vi "Tx Message to Map Value.vi"(7 "parameter index":i32, 8 "error in":errorcluster, 9 "message":T2={"name"="", "message type"="BC to RT", "endpoint Tx"={"terminal address"=0, "subaddress"=0}, "endpoint Rx"={"terminal address"=0, "subaddress"=0}, "create timestamp channel"=FALSE, "mode code"=0, "number of words"=0, "parameters"=[]}, 10 "remote terminal handles":u64[](array[numeric]), 11 "bus controller handle":u64) -> (0 "error out":errorcluster, 3 "Tx write info":T1, 5 "next parameter index":i32)   [LabVIEW 2020, in "Ballard MIL-STD-1553 Engine.lvlib" / "Custom Device.lvlib"]
uses:
  Custom Device.lvlib
  Shared/Message Definition.ctl
  Shared/Message Type.ctl
  Shared/Terminal Endpoint.ctl
  Shared/Address.ctl
  Shared/Parameter Definition.ctl
  Shared/Tx Write Info.ctl
  <instrlib>/BTI1553Lib/Public/Controls/1553 RT Transfer Type.ctl
  <instrlib>/BTI1553Lib/Public/Controls/1553 Transfer Direction.ctl
  <instrlib>/BTI1553Lib/Private/RT/Configure/Get RT Xfer Handle.vi
  <instrlib>/BTI1553Lib/BTI1553LV.lvlib
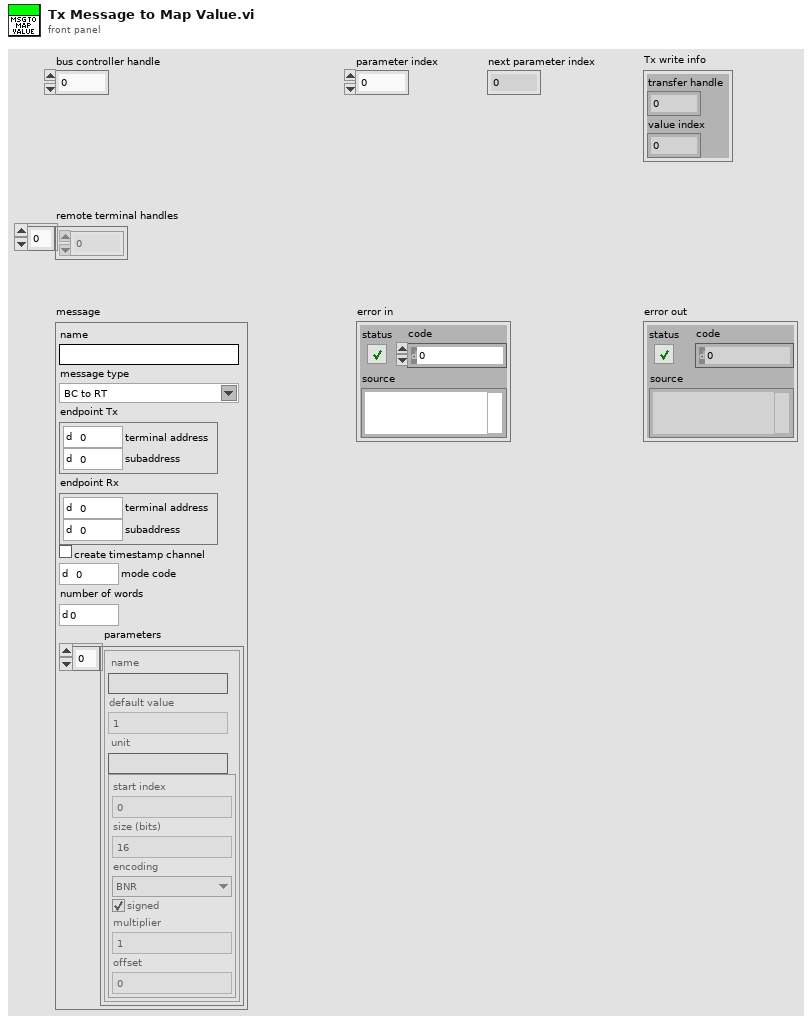
[diagram p1: front panel]
types:
  T1 = typedef "Tx Write Info.ctl" = cluster{"transfer handle":u64, "value index":i32}
  T2 = typedef "Message Definition.ctl" = cluster{"name":string, "message type":T3, "endpoint Tx":T4, "endpoint Rx":T4, "create timestamp channel":bool, "mode code":u16, "number of words":u16, "parameters":cluster{"name":string, "default value":dbl, "unit":string, "parameter definition":T6}[]}
  T3 = typedef "Message Type.ctl" = string
  T4 = typedef "Terminal Endpoint.ctl" = cluster{"terminal address":T5, "subaddress":T5}
  T5 = typedef "Address.ctl" = u16
  T6 = typedef "Parameter Definition.ctl" = cluster{"start index":i32, "size (bits)":i32, "encoding":enum16{"BNR", "BCD", "Discrete"}, "signed":bool, "multiplier":dbl, "offset":dbl}
  T7 = typedef "BTI1553LV.lvlib/1553 Transfer Direction.ctl" = u32
  T8 = typedef "BTI1553LV.lvlib/1553 RT Transfer Type.ctl" = u32
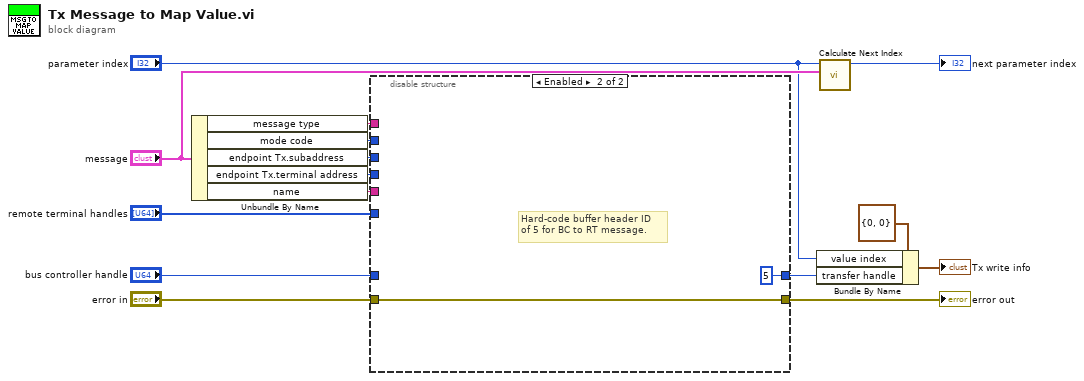
[diagram p0: block diagram]
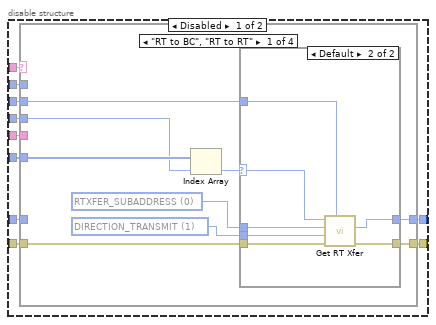
[diagram p2: hidden frame]
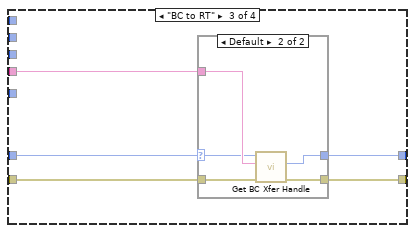
[diagram p5: hidden frame]
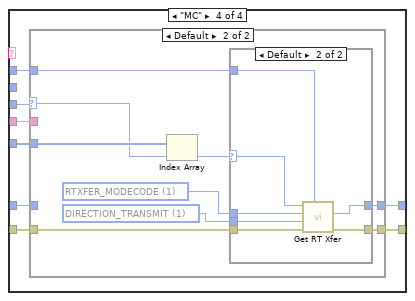
[diagram p7: hidden frame]
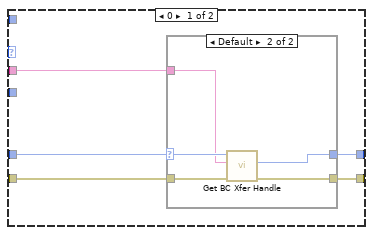
[diagram p8: hidden frame]
diagram:
  n1 = Unbundle By Name("message") -> ("message type"=w1:T3, "mode code"=w8:u16, "endpoint Tx.subaddress"=w15:T5, "endpoint Tx.terminal address"=w14:T5, "name"=w2:string)
  n2 = disable-structure shown="Enabled" {
    disable-tunnel: w15 -> [w25 _]
    disable-tunnel: w14 -> [w24 _]
    disable-tunnel: w8 -> [w23 _]
    disable-tunnel: "error in" -> [w22 w92]
    disable-tunnel: "remote terminal handles" -> [w21 _]
    disable-tunnel: [w20 u64 5 ("rt transfer handle out")] -> w5
    disable-tunnel: [w19 w92] -> w4
    disable-tunnel: "bus controller handle" -> [w18 _]
    disable-tunnel: w2 -> [w17 _]
    disable-tunnel: w1 -> [w16 _]
    frame Disabled {
      n3 = case shown="\"RT to BC\", \"RT to RT\"" w16 {
        tunnel: w25 -> [w27 _ _ _]
        tunnel: w24 -> [w26 _ _ w62]
        tunnel: w23 -> [_ _ _ w58]
        tunnel: w22 -> [w34 w43 w45 w61]
        tunnel: w21 -> [w31 _ _ w59]
        tunnel: [w29 _ w48 w57] -> w20
        tunnel: [w28 w43 w44 w60] -> w19
        tunnel: w18 -> [_ _ w46 w56]
        tunnel: w17 -> [_ _ w47 w55]
        frame "RT to BC", "RT to RT" {
          w33 = T7 1 items=["DIRECTION_RECEIVE", "DIRECTION_TRANSMIT"] ("transfer direction")
          w32 = T8 0 items=["RTXFER_SUBADDRESS", "RTXFER_MODECODE"] ("transfer type")
          n4 = Index Array(array=w31, index=w26) -> (element=w30:u64)
          n5 = case shown="Default" w30 {
            selector: w30 -> [_ w39]
            tunnel: w34 -> [w35 w42]
            tunnel: w33 -> [_ w41]
            tunnel: w32 -> [_ w40]
            tunnel: [_ w38] -> w29
            tunnel: [w35 w37] -> w28
            tunnel: w27 -> [_ w36]
            frame 0, -1 {
            }
            frame Default {
              n6 = call-poly <instrlib>:"Get RT Xfer.vi"("transfer sa number or mc number"=w36, "error in (no error)"=w42, "transfer direction"=w41, "transfer type"=w40, "remote terminal handle in"=w39) -> ("error out"=w37:errorcluster, "rt transfer handle out"=w38:u64)  [unwired: 4 in, 1 out]
            }
          }
        }
        frame Default {
        }
        frame "BC to RT" {
          n7 = case shown="Default" w46 {
            selector: w46 -> [_ w52]
            tunnel: [_ w54] -> w48
            tunnel: w47 -> [_ w53]
            tunnel: w45 -> [w49 w51]
            tunnel: [w49 w50] -> w44
            frame 0, -1 {
            }
            frame Default {
              n8 = call <instrlib>:"Get BC Xfer Handle.vi"("error in (no error)"=w51, "bc transfer name"=w53, "bus controller handle in"=w52) -> ("error out"=w50:errorcluster, "bc transfer handle out"=w54:u64)  [unwired: 6 in, 1 out]
            }
          }
        }
        frame "MC" {
          n9 = case shown="Default" w62 {
            selector: w62 -> [_ w77]
            tunnel: w61 -> [w67 w82]
            tunnel: [w66 w81] -> w60
            tunnel: w59 -> [_ w78]
            tunnel: w58 -> [_ w75]
            tunnel: [w63 w74] -> w57
            tunnel: w56 -> [w65 _]
            tunnel: w55 -> [w64 _]
            frame 0 {
              n10 = case shown="Default" w65 {
                selector: w65 -> [_ w71]
                tunnel: w67 -> [w68 w73]
                tunnel: [w68 w72] -> w66
                tunnel: w64 -> [_ w70]
                tunnel: [_ w69] -> w63
                frame 0, -1 {
                }
                frame Default {
                  n11 = call <instrlib>:"Get BC Xfer Handle.vi"("error in (no error)"=w73, "bc transfer name"=w70, "bus controller handle in"=w71) -> ("error out"=w72:errorcluster, "bc transfer handle out"=w69:u64)  [unwired: 6 in, 1 out]
                }
              }
            }
            frame Default {
              w79 = T8 1 items=["RTXFER_SUBADDRESS", "RTXFER_MODECODE"] ("transfer type")
              w80 = T7 1 items=["DIRECTION_RECEIVE", "DIRECTION_TRANSMIT"] ("transfer direction")
              n12 = Index Array(array=w78, index=w77) -> (element=w76:u64)
              n13 = case shown="Default" w76 {
                selector: w76 -> [_ w86]
                tunnel: w82 -> [w83 w90]
                tunnel: [w83 w89] -> w81
                tunnel: w80 -> [_ w88]
                tunnel: w79 -> [_ w87]
                tunnel: w75 -> [_ w85]
                tunnel: [_ w84] -> w74
                frame 0, -1 {
                }
                frame Default {
                  n14 = call-poly <instrlib>:"Get RT Xfer.vi"("transfer sa number or mc number"=w85, "error in (no error)"=w90, "transfer direction"=w88, "transfer type"=w87, "remote terminal handle in"=w86) -> ("error out"=w89:errorcluster, "rt transfer handle out"=w84:u64)  [unwired: 4 in, 1 out]
                }
              }
            }
          }
        }
      }
    }
    frame Enabled {
      # "Hard-code buffer header ID\nof 5 for BC to RT message."
    }
  }
  "error out" <- w4
  n15 = Bundle By Name(cluster=T1 {"transfer handle"=0, "value index"=0} ("Tx write info"), "value index"="parameter index", "transfer handle"=w5) -> (→"Tx write info":T1)
  n16 = call "Calculate Next Index.vi"("message"="message", "index"="parameter index") -> ("next index"=→"next parameter index":i32)  [unwired: 9 in]
